vi "Check_C1C2_detector.vi"(11 "File name":string) -> (3 "Detector":u16, 5 "Frame number":i32)   [LabVIEW 2022 SP3]
panel:
  out "offset past match 2":i32
  out "offset past match":i32
  out "substring":string
  # "\"-1\"  -- no detector identified (failure)\n\"0\" -- detector 1 , YJ  = C0 \n\"1\"- - detector 2, HK = C1"
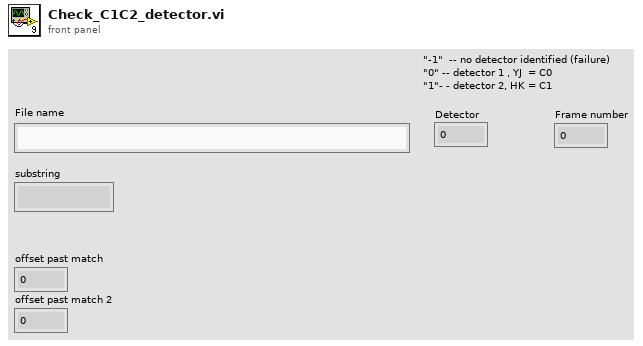
[diagram p1: front panel]
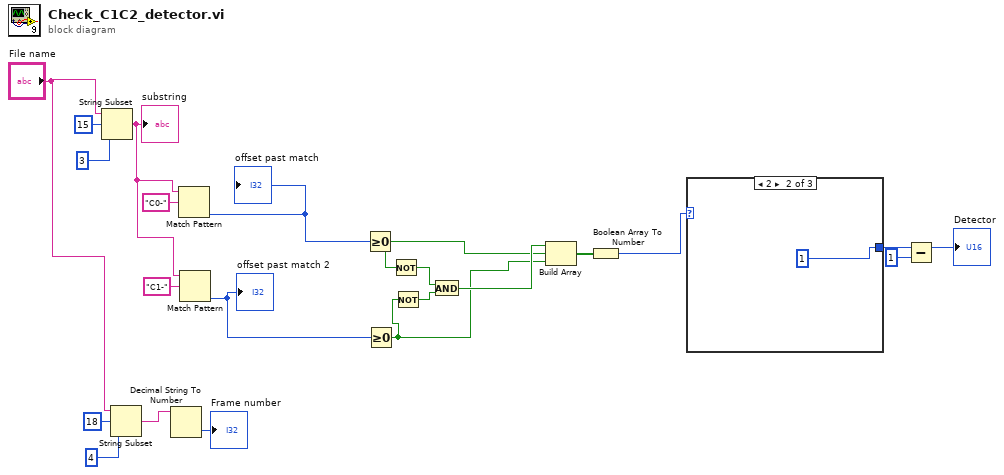
[diagram p0: block diagram]
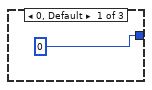
[diagram p2: hidden frame]
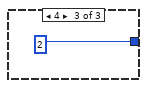
[diagram p3: hidden frame]
diagram:
  n1 = String Subset(string="File name", offset (0)=15, length (rest)=3 ("length (rest)")) -> (substring=w18:string)
  "substring" <- w18
  n2 = String Subset(string="File name", offset (0)=18, length (rest)=4 ("length (rest)")) -> (substring=w4:string)
  n3 = Decimal String To Number(string=w4) -> (number=→"Frame number":i32)  [unwired: 2 in, 1 out]
  n4 = Match Pattern(string=w18, regular expression="C0-") -> (offset past match=w17:i32)  [unwired: 1 in, 3 out]
  "offset past match" <- w17
  n5 = Match Pattern(string=w18, regular expression="C1-") -> (offset past match=w16:i32)  [unwired: 1 in, 3 out]
  "offset past match 2" <- w16
  n6 = Greater Or Equal To 0?(x=w17) -> (x >= 0?=w12:bool)
  n7 = Greater Or Equal To 0?(x=w16) -> (x >= 0?=w11:bool)
  n8 = Not(x=w12) -> (.not. x?=w14:bool)
  n9 = Not(x=w11) -> (.not. x?=w15:bool)
  n10 = And(x=w14, y=w15) -> (x .and. y?=w13:bool)
  n11 = Build Array(w13, w12, w11) -> (w10:bool[])
  n12 = Boolean Array To Number(Boolean array=w10) -> (number=w9:u32)
  n13 = case shown="2" w9 {
    tunnel: [0 1 2] -> w8
    frame 0, Default {
    }
    frame 2 {
    }
    frame 4 {
    }
  }
  n14 = Subtract(x=w8, y=1) -> (x-y=→"Detector":i32)
